vi "Mouse Down.vi"(8 "error in (no error)":errorcluster, 10 "Delay in ms (10)":u32=10, 11 "Right Click? (F)":bool) -> (0 "error out":errorcluster)   [LabVIEW 2023]
uses:
  fdaed37b-1ab6-437a-8e89-3a5b05fa2717.vi
  User32.dll
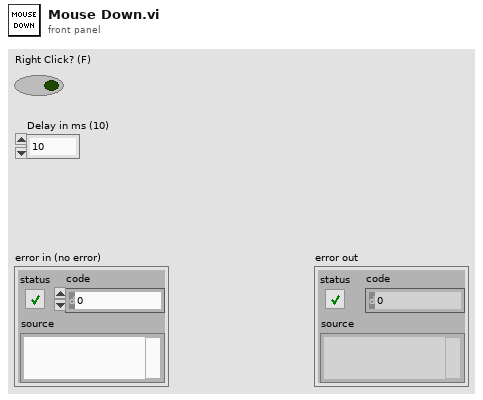
[diagram p1: front panel]
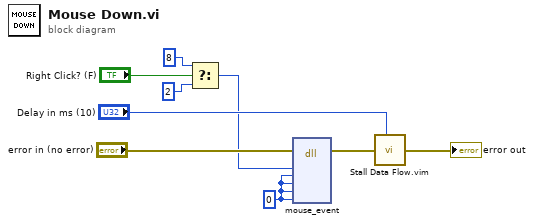
[diagram p0: block diagram]
diagram:
  w9 = 0 ("dx")
  n1 = Select(t=8 ("y"), s="Right Click? (F)", f=2 ("y")) -> (s? t:f=w1:i32)
  n2 = dll-call lib="user32.dll" fn="mouse_event"(error in="error in (no error)", "flags"=w1, "dx"=w9, "dx"=w9, "data"=w9, "ptr"=w9) -> (error out=w6:errorcluster)  [unwired: 8 in, 1 out]
  n3 = call "Stall Data Flow.vim"("value in"=w6, "milliseconds to wait"="Delay in ms (10)") -> ("value out"=→"error out":errorcluster)  [unwired: 1 out]
